vi "Close.vi"(2 "error in":errorcluster, 3 "VISA arduino in":refnum<visa-resource-name>) -> (0 "error out":errorcluster)   [LabVIEW 2021]
uses:
  <vilib>/Utility/error.llb/Error Cluster From Error Code.vi
  <vilib>/ErrorRing/Error Ring.xnode
panel:
  out "delay":u32
  # "Private"
  # "Public"
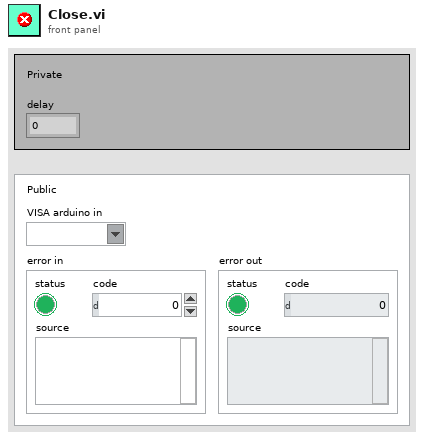
[diagram p1: front panel]
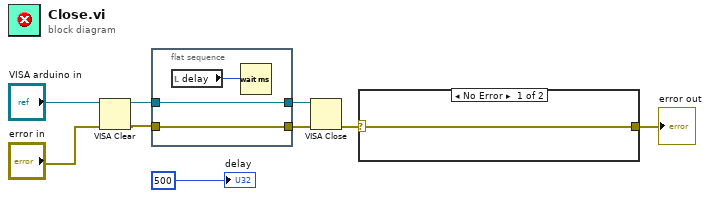
[diagram p0: block diagram]
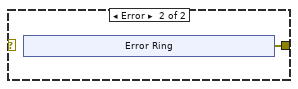
[diagram p2: hidden frame]
diagram:
  n1 = VISA Clear(VISA resource name="VISA arduino in", error in (no error)="error in") -> (VISA resource name out=w7:refnum<visa-resource-name>, error out=w8:errorcluster)
  n2 = flat-sequence {
    tunnel: [w12] -> w5
    tunnel: w7 -> [w12]
    tunnel: [w11] -> w6
    tunnel: w8 -> [w11]
    frame #0 {
      n3 = local read "delay"() -> (w10:u32)
      n4 = Wait (ms)(milliseconds to wait=w10) -> ()  [unwired: 1 out]
    }
  }
  n5 = VISA Close(VISA resource name=w5, error in (no error)=w6) -> (error out=w4:errorcluster)
  n6 = case shown="No Error" w4 {
    selector: w4 -> [w13 _]
    tunnel: [w13 w14] -> w3
    frame No Error {
    }
    frame Error {
      n7 = xnode "Error Ring"() -> ("error out"=w14:errorcluster)
    }
  }
  "error out" <- w3
  "delay" <- u32 500
